vi "writeToXML.vi"(8 "error in (no error)":errorcluster, 10 "Class Label":string="CurrentRotatorPositions", 11 "CurrentRotatorPositions in":refnum<class "CurrentRotatorPositions.lvclass">) -> (0 "error out":errorcluster, 2 "XML out":string="<>\n  <iaa>0</iaa>\n  <rotIPD>0</rotIPD>\n</>", 3 "CurrentRotatorPositions out":refnum<class "CurrentRotatorPositions.lvclass">)   [LabVIEW 2022 SP3, in "TCSDataDefinitions.lvlib" / "TCSPublicStatus.lvlib" / "PointingPositions.lvlib" / "CurrentRotatorPositions.lvclass"]
uses:
  CurrentRotatorPositions.lvclass
  <userlib>/Common/UnitsAndXML/FlattenItemWithUnitToXML/FlattenPlaneAngleToXML/PlaneAngleUnit.ctl
  CurrentRotatorPositions.lvclass/CurrentRotatorPositions.ctl
  RotatorPositions/RotatorPositions.lvclass
  <userlib>/Common/UnitsAndXML/UnitsAndXML.lvlib
  <userlib>/Common/XML/XMLGenerator/XMLGenerator.lvclass
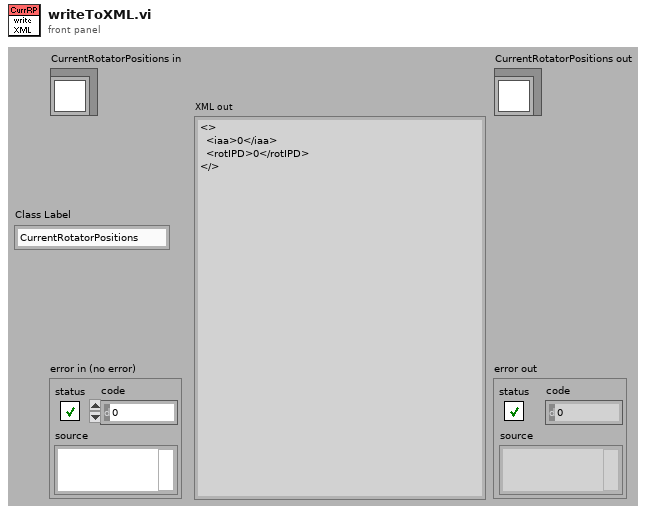
[diagram p1: front panel]
types:
  T1 = typedef "UnitsAndXML.lvlib/PlaneAngleUnit.ctl" = enum16{"rad", "deg", "'", "\""}
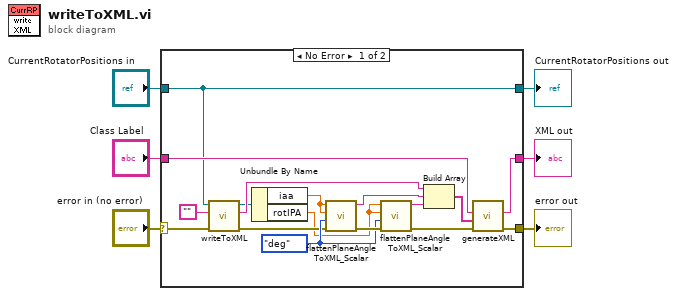
[diagram p0: block diagram]
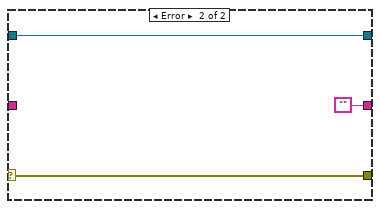
[diagram p2: hidden frame]
diagram:
  n1 = case shown="No Error" "error in (no error)" {
    selector: "error in (no error)" -> [w14 w26]
    tunnel: [w19 w26] -> w5
    tunnel: [w9 w25] -> w3
    tunnel: "CurrentRotatorPositions in" -> [w9 w25]
    tunnel: "Class Label" -> [w15 _]
    tunnel: [w20 ""] -> w1
    frame No Error {
      w16 = PlaneAngleUnit."deg" ("planeAngleUnitInXML")
      n2 = call-parent "writeToXML.vi"("error in (no error)"=w14, "Class Label"="", "RotatorPositions in"=w9) -> ("error out"=w13:errorcluster, "XML out"=w12:string, "RotatorPositions out"=w8:refnum<class "CurrentRotatorPositions.lvclass">)  [unwired: 6 in]
      n3 = Unbundle By Name(w8) -> ("iaa"=w11:dbl[unit], "rotIPA"=w10:dbl[unit])
      n4 = call <userlib>:"flattenPlaneAngleToXML_Scalar.vi"("error in (no error)"=w13, "planeAngleUnitInXML"=w16, "planeAngleAgain"=w11, "planeAngle"=w11) -> ("error out"=w17:errorcluster, "xmlString"=w23:string)  [unwired: 6 in]
      n5 = call <userlib>:"flattenPlaneAngleToXML_Scalar.vi"("error in (no error)"=w17, "planeAngleUnitInXML"=w16, "planeAngleAgain"=w10, "planeAngle"=w10) -> ("error out"=w18:errorcluster, "xmlString"=w22:string)  [unwired: 6 in]
      n6 = Build Array(w12, w23, w22) -> (w21:string[])
      n7 = call <userlib>:"generateXML.vi"("error in"=w18, "childrenXML"=w21, "elementName"=w15) -> ("error out"=w19:errorcluster, "XML out"=w20:string)  [unwired: 6 in, 1 out]
    }
    frame Error {
    }
  }
  "error out" <- w5
  "CurrentRotatorPositions out" <- w3
  "XML out" <- w1
